vi "Value To Audio Device Refnum.vi"(11 "Refnum Value":i32) -> (3 "Audio Device Refnum":T1)   [LabVIEW 2020, in "G-Audio.lvlib"]
uses:
  Controls/Audio Device Refnum.ctl
  G-Audio.lvlib
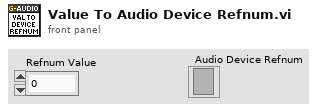
[diagram p1: front panel]
types:
  T1 = typedef "G-Audio.lvlib/Audio Device Refnum.ctl" = refnum<file>
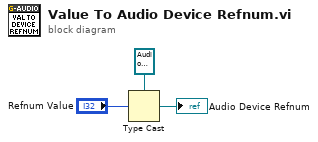
[diagram p0: block diagram]
diagram:
  n1 = Type Cast(type=T1 refnum ("Audio Device Refnum"), x="Refnum Value") -> (*(type *) &x=→"Audio Device Refnum":T1)
